vi "CursorKinGraphMove.vi"(8 "error in (no error)":errorcluster, 9 "change":bool, 10 "Clean mode":enum32{"delete", "approx"}(radio)=enum."approx", 11 "Control-Client in":refnum<class "Control-Client.lvclass">) -> (0 "error out":errorcluster, 3 "Control-Client out":refnum<class "Control-Client.lvclass">)   [LabVIEW 2018, in "Control-Client.lvclass"]
uses:
  Control-Client.lvclass
  Control-Client.lvclass/Control-Client.ctl
  Experiments/Experiment.lvclass
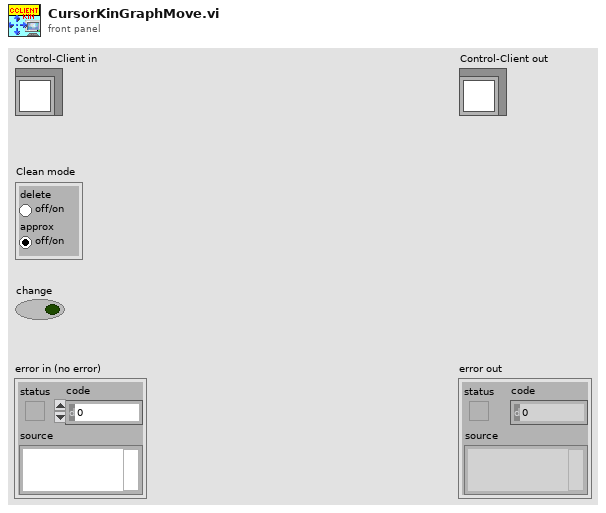
[diagram p1: front panel]
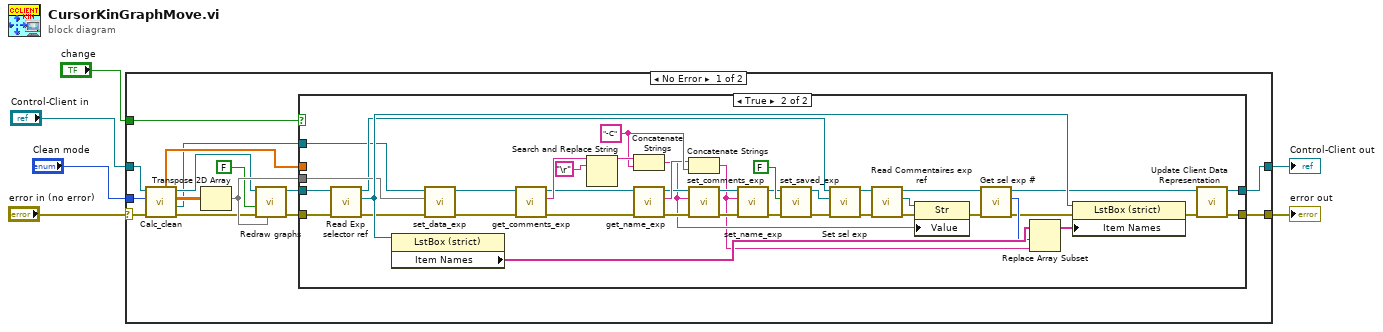
[diagram p0: block diagram]
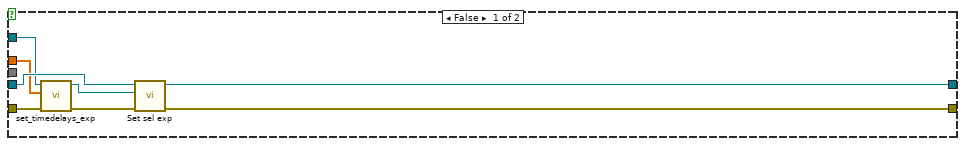
[diagram p2: hidden frame]
diagram:
  n1 = case shown="No Error" "error in (no error)" {
    selector: "error in (no error)" -> [w19 w72]
    tunnel: [w8 w72] -> w5
    tunnel: [w9 w71] -> w3
    tunnel: "Control-Client in" -> [w16 w71]
    tunnel: "Clean mode" -> [w20 _]
    tunnel: "change" -> [w13 _]
    frame No Error {
      n2 = call "Calc_clean.vi"("error in (no error)"=w19, "Clean mode"=w20, "Control-Client in"=w16) -> ("error out"=w11:errorcluster, "Experiment.lvclass out"=w7:refnum<class "Experiment.lvclass">, "Data out"=w21:dbl[][], "Control-Client out"=w12:refnum<class "Control-Client.lvclass">, "timedelays old"=w10:dbl[])  [unwired: 4 in]
      n3 = Transpose 2D Array(2D array=w21) -> (transposed array=w15:dbl[][])
      n4 = call "Redraw graphs.vi"("Data"=w15, "error in (no error)"=w11, "Selected exp"=FALSE, "Control-Client in"=w12) -> ("error out"=w17:errorcluster, "Control-Client out"=w18:refnum<class "Control-Client.lvclass">)  [unwired: 6 in]
      n5 = case shown="True" w13 {
        tunnel: w18 -> [w26 w70]
        tunnel: w17 -> [w29 w69]
        tunnel: [w25 w30] -> w9
        tunnel: [w24 w33] -> w8
        tunnel: w15 -> [_ w37]
        tunnel: w7 -> [w23 w34]
        tunnel: w10 -> [w22 _]
        frame False {
          n6 = call "set_timedelays_exp.vi"("error in (no error)"=w29, "timedelays"=w22, "Experiment.lvclass in"=w23) -> ("error out"=w28:errorcluster, "Experiment.lvclass out"=w27:refnum<class "Experiment.lvclass">)  [unwired: 7 in]
          n7 = call "Set sel exp.vi"("error in (no error)"=w28, "Experiment"=w27, "Control-Client in"=w26) -> ("error out"=w24:errorcluster, "Control-Client out"=w25:refnum<class "Control-Client.lvclass">)  [unwired: 7 in]
        }
        frame True {
          w60 = "-C" ("string")
          n8 = call "Read Exp selector ref.vi"("error in (no error)"=w69, "Control-Client in"=w70) -> ("error out"=w35:errorcluster, "Exp selector ref"=w63:refnum<vi>, "Control-Client out"=w36:refnum<class "Control-Client.lvclass">)  [unwired: 7 in]
          n9 = property on="Property Node" class="LstBox (strict)"(reference=w63) -> ("Item Names"=w62:string[])  [unwired: 1 in, 2 out]
          n10 = call "set_data_exp.vi"("error in (no error)"=w35, "Data"=w37, "Experiment.lvclass in"=w34) -> ("error out"=w49:errorcluster, "Experiment.lvclass out"=w52:refnum<class "Experiment.lvclass">)  [unwired: 7 in]
          n11 = call "get_comments_exp.vi"("error in (no error)"=w49, "Experiment.lvclass in"=w52) -> ("error out"=w54:errorcluster, "Comments"=w67:string, "Experiment.lvclass out"=w51:refnum<class "Experiment.lvclass">)  [unwired: 7 in]
          n12 = Search and Replace String(input string=w67, search string="\r") -> (result string=w68:string)  [unwired: 6 in, 3 out]
          n13 = Concatenate Strings(w68, w60) -> (w41:string)
          n14 = call "get_name_exp.vi"("error in (no error)"=w54, "Experiment.lvclass in"=w51) -> ("error out"=w53:errorcluster, "Exp name"=w55:string, "Experiment.lvclass out"=w50:refnum<class "Experiment.lvclass">)  [unwired: 7 in]
          n15 = Concatenate Strings(w55, w60) -> (w40:string)
          n16 = call "set_comments_exp.vi"("error in (no error)"=w53, "Comments"=w41, "Experiment.lvclass in"=w50) -> ("error out"=w57:errorcluster, "Experiment.lvclass out"=w56:refnum<class "Experiment.lvclass">)  [unwired: 7 in]
          n17 = call "set_name_exp.vi"("error in (no error)"=w57, "Exp name"=w40, "Experiment.lvclass in"=w56) -> ("error out"=w59:errorcluster, "Experiment.lvclass out"=w58:refnum<class "Experiment.lvclass">)  [unwired: 7 in]
          n18 = call "set_saved_exp.vi"("error in (no error)"=w59, "Saved"=FALSE, "Experiment.lvclass in"=w58) -> ("error out"=w38:errorcluster, "Experiment.lvclass out"=w39:refnum<class "Experiment.lvclass">)  [unwired: 7 in]
          n19 = call "Set sel exp.vi"("error in (no error)"=w38, "Experiment"=w39, "Control-Client in"=w36) -> ("error out"=w65:errorcluster, "Control-Client out"=w64:refnum<class "Control-Client.lvclass">)  [unwired: 7 in]
          n20 = call "Read Commentaires exp ref.vi"("error in (no error)"=w65, "Control-Client in"=w64) -> ("error out"=w45:errorcluster, "Commentaires exp ref"=w46:refnum<vi>, "Control-Client out"=w44:refnum<class "Control-Client.lvclass">)  [unwired: 7 in]
          n21 = property on="Property Node" class="Str"(reference=w46, error in=w45, "Value"=w41) -> (error out=w43:errorcluster)  [unwired: 1 out]
          n22 = call "Get sel exp #.vi"("error in (no error)"=w43, "Control-Client in"=w44) -> ("error out"=w42:errorcluster, "Exp sel #"=w47:i32, "Control-Client out"=w32:refnum<class "Control-Client.lvclass">)  [unwired: 7 in]
          n23 = Replace Array Subset(array=w62, new element=w40, index=w47) -> (w48:string[])
          n24 = property on="Property Node" class="LstBox (strict)"(reference=w63, error in=w42, "Item Names"=w48) -> (error out=w31:errorcluster)  [unwired: 1 out]
          n25 = call "Update Client Data Representation.vi"("error in (no error)"=w31, "Control-Client in"=w32) -> ("error out"=w33:errorcluster, "Control-Client out"=w30:refnum<class "Control-Client.lvclass">)  [unwired: 8 in]
        }
      }
    }
    frame Error {
    }
  }
  "error out" <- w5
  "Control-Client out" <- w3
